vi "Read Values.vi"(7 "Force rev":bool, 8 "error in (no error)":errorcluster, 10 "string":string) -> (0 "error out":errorcluster, 2 "Read values":T1, 3 "Array":string[](array[string]))   [LabVIEW 2019, in "STAV lib.lvlib"]
uses:
  STAV lib.lvlib
  Read Values.ctl
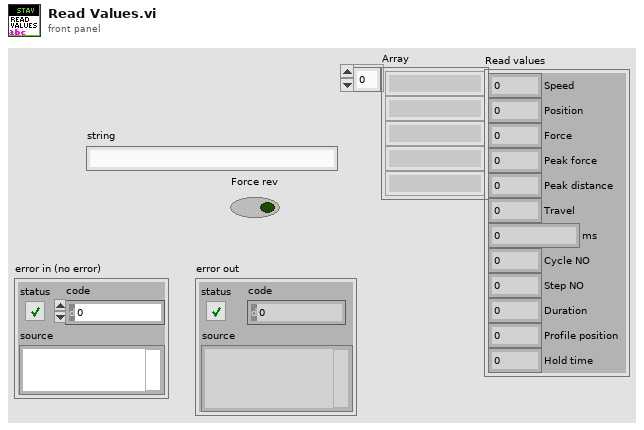
[diagram p1: front panel]
types:
  T1 = typedef "STAV lib.lvlib/Read Values.ctl" = cluster{"Speed":dbl, "Position":dbl, "Force":dbl, "Peak force":dbl, "Peak distance":dbl, "Travel":dbl, "ms":u32, "Cycle NO":dbl, "Step NO":dbl, "Duration":dbl, "Profile position":dbl, "Hold time":dbl}
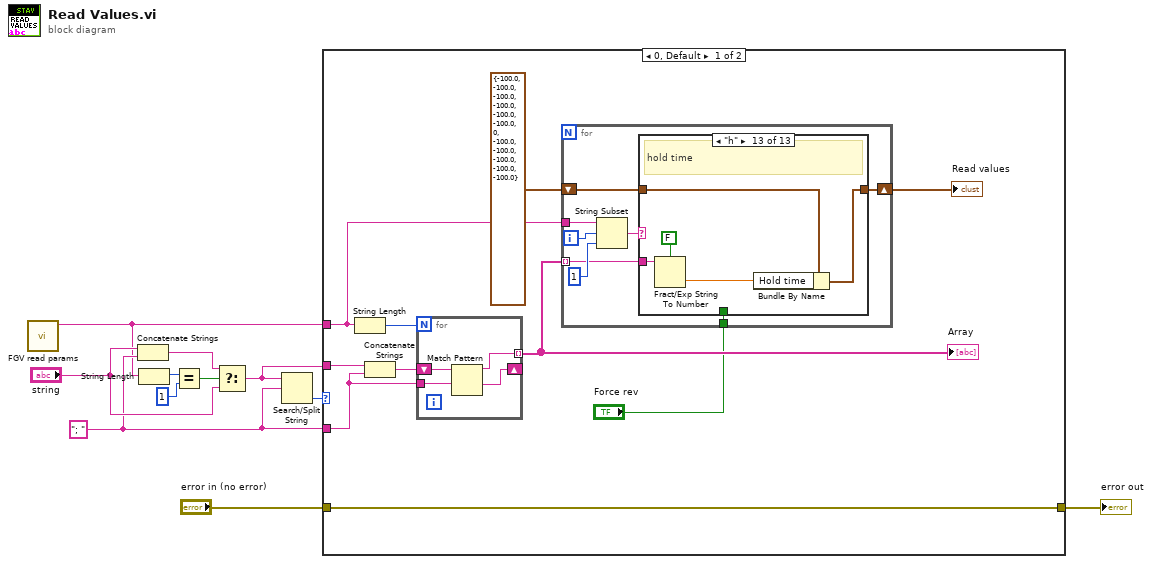
[diagram p0: block diagram]
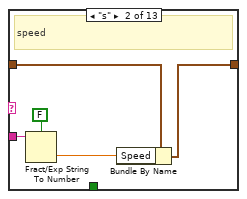
[diagram p3: hidden frame]
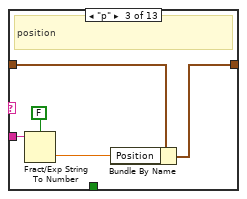
[diagram p4: hidden frame]
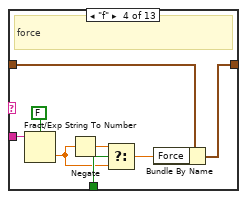
[diagram p5: hidden frame]
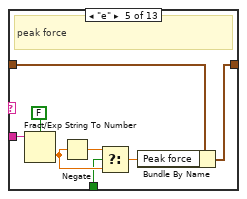
[diagram p6: hidden frame]
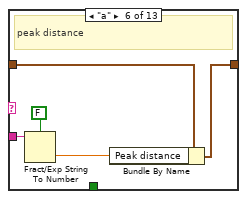
[diagram p7: hidden frame]
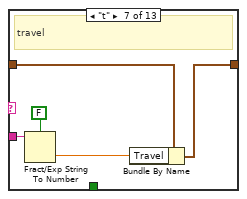
[diagram p8: hidden frame]
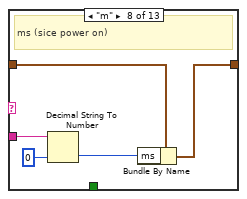
[diagram p9: hidden frame]
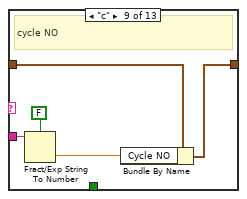
[diagram p10: hidden frame]
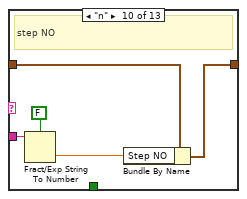
[diagram p11: hidden frame]
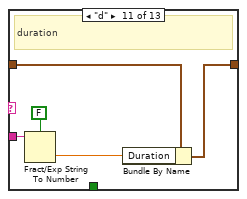
[diagram p12: hidden frame]
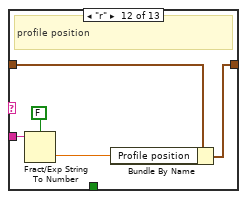
[diagram p13: hidden frame]
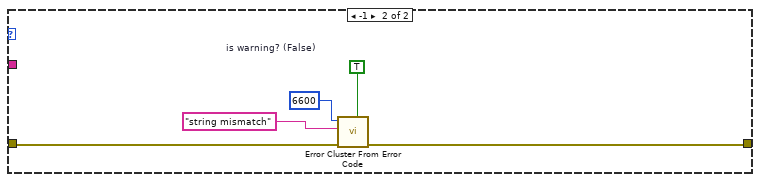
[diagram p14: hidden frame]
diagram:
  w2 = "; " ("string")
  n1 = call "FGV read params.vi"() -> ("params out"=w1:string)  [unwired: 11 in]
  n2 = Concatenate Strings("string", w2) -> (w4:string)
  n3 = String Length(string=w1) -> (length=w8:i32)
  n4 = Equal?(x=w8, y=1) -> (x = y?=w6:bool)
  n5 = Select(t=w4, s=w6, f="string") -> (s? t:f=w3:string)
  n6 = Search/Split String(string=w3, search string/char (-)=w2) -> (offset of match=w9:i32)  [unwired: 1 in, 2 out]
  n7 = case shown="0, Default" w9 {
    tunnel: w1 -> [w19 _]
    tunnel: w3 -> [w15 _]
    tunnel: w2 -> [w14 _]
    tunnel: "error in (no error)" -> [w13 w105]
    tunnel: [w13 w104] -> w10
    frame 0, Default {
      n8 = String Length(string=w19) -> (length=w21:i32)
      n9 = Concatenate Strings(w15, w14) -> (w20:string)
      n10 = for {
        N: w21 -> [_]
        shift-right: [w99] -> _
        shift-left: w20 -> [w100]
        tunnel: [w98] -> w18 mode=indexing
        tunnel: w14 -> [w97]
        n11 = Match Pattern(string=w100, regular expression=w97) -> (before substring=w98:string, after substring=w99:string)  [unwired: 1 in, 2 out]
      }
      "Array" <- w18
      n12 = for {
        tunnel: w19 -> [w28]
        tunnel: w18 -> [w23] mode=indexing
        shift-right: [w24] -> w16
        shift-left: T1 {"Speed"=-100.0, "Position"=-100.0, "Force"=-100.0, "Peak force"=-100.0, "Peak distance"=-100.0, "Travel"=-100.0, "ms"=0, "Cycle NO"=-100.0, "Step NO"=-100.0, "Duration"=-100.0, "Profile position"=-100.0, "Hold time"=-100.0} ("Read values") -> [w25]
        tunnel: "Force rev" -> [w22]
        i -> [w29]
        n13 = String Subset(string=w28, offset (0)=w29, length (rest)=1 ("length (rest)")) -> (substring=w26:string)
        n14 = case shown="\"h\"" w26 {
          tunnel: w25 -> [w30 w35 w40 w48 w56 w61 w66 w71 w76 w81 w86 w91 w96]
          tunnel: [w30 w34 w39 w47 w55 w60 w65 w70 w75 w80 w85 w90 w95] -> w24
          tunnel: w23 -> [_ w31 w36 w45 w53 w57 w62 w69 w72 w77 w82 w87 w92]
          tunnel: w22 -> [_ _ _ w43 w49 _ _ _ _ _ _ _ _]
          frame "False", Default {
          }
          frame "s" {
            # "speed"
            n15 = Fract/Exp String To Number(use system decimal point (T)=FALSE, string=w31) -> (number=w33:dbl)  [unwired: 2 in, 1 out]
            n16 = Bundle By Name(cluster=w35, "Speed"=w33) -> (w34:T1)
          }
          frame "p" {
            # "position"
            n17 = Fract/Exp String To Number(use system decimal point (T)=FALSE, string=w36) -> (number=w38:dbl)  [unwired: 2 in, 1 out]
            n18 = Bundle By Name(cluster=w40, "Position"=w38) -> (w39:T1)
          }
          frame "f" {
            # "force"
            n19 = Fract/Exp String To Number(use system decimal point (T)=FALSE, string=w45) -> (number=w41:dbl)  [unwired: 2 in, 1 out]
            n20 = Negate(x=w41) -> (-x=w42:dbl)
            n21 = Select(t=w42, s=w43, f=w41) -> (s? t:f=w44:dbl)
            n22 = Bundle By Name(cluster=w48, "Force"=w44) -> (w47:T1)
          }
          frame "e" {
            # "peak force"
            n23 = Fract/Exp String To Number(use system decimal point (T)=FALSE, string=w53) -> (number=w51:dbl)  [unwired: 2 in, 1 out]
            n24 = Negate(x=w51) -> (-x=w52:dbl)
            n25 = Select(t=w52, s=w49, f=w51) -> (s? t:f=w50:dbl)
            n26 = Bundle By Name(cluster=w56, "Peak force"=w50) -> (w55:T1)
          }
          frame "a" {
            # "peak distance"
            n27 = Fract/Exp String To Number(use system decimal point (T)=FALSE, string=w57) -> (number=w59:dbl)  [unwired: 2 in, 1 out]
            n28 = Bundle By Name(cluster=w61, "Peak distance"=w59) -> (w60:T1)
          }
          frame "t" {
            # "travel"
            n29 = Fract/Exp String To Number(use system decimal point (T)=FALSE, string=w62) -> (number=w64:dbl)  [unwired: 2 in, 1 out]
            n30 = Bundle By Name(cluster=w66, "Travel"=w64) -> (w65:T1)
          }
          frame "m" {
            # "ms (sice power on)"
            n31 = Decimal String To Number(string=w69, default (0L)=u32 0) -> (number=w68:u32)  [unwired: 1 in, 1 out]
            n32 = Bundle By Name(cluster=w71, "ms"=w68) -> (w70:T1)
          }
          frame "c" {
            # "cycle NO"
            n33 = Fract/Exp String To Number(use system decimal point (T)=FALSE, string=w72) -> (number=w74:dbl)  [unwired: 2 in, 1 out]
            n34 = Bundle By Name(cluster=w76, "Cycle NO"=w74) -> (w75:T1)
          }
          frame "n" {
            # "step NO"
            n35 = Fract/Exp String To Number(use system decimal point (T)=FALSE, string=w77) -> (number=w79:dbl)  [unwired: 2 in, 1 out]
            n36 = Bundle By Name(cluster=w81, "Step NO"=w79) -> (w80:T1)
          }
          frame "d" {
            # "duration"
            n37 = Fract/Exp String To Number(use system decimal point (T)=FALSE, string=w82) -> (number=w84:dbl)  [unwired: 2 in, 1 out]
            n38 = Bundle By Name(cluster=w86, "Duration"=w84) -> (w85:T1)
          }
          frame "r" {
            # "profile position"
            n39 = Fract/Exp String To Number(use system decimal point (T)=FALSE, string=w87) -> (number=w89:dbl)  [unwired: 2 in, 1 out]
            n40 = Bundle By Name(cluster=w91, "Profile position"=w89) -> (w90:T1)
          }
          frame "h" {
            # "hold time"
            n41 = Fract/Exp String To Number(use system decimal point (T)=FALSE, string=w92) -> (number=w94:dbl)  [unwired: 2 in, 1 out]
            n42 = Bundle By Name(cluster=w96, "Hold time"=w94) -> (w95:T1)
          }
        }
      }
      "Read values" <- w16
    }
    frame -1 {
      w103 = TRUE  # is warning? (False)
      n43 = call <vilib>:"Error Cluster From Error Code.vi"("is warning? (False)"=w103, "error in (no error)"=w105, "error message (\"\")"="string mismatch" ("error message (\"\")"), "error code (0)"=6600) -> ("error out"=w104:errorcluster)  [unwired: 5 in]
    }
  }
  "error out" <- w10
